vi "Error Handler.vi"(8 "error in":errorcluster, 11 "Engine in":refnum<class "Engine.lvclass">) -> (0 "error out":errorcluster, 2 "Stop Application":bool, 3 "Engine out":refnum<class "Engine.lvclass">)   [LabVIEW 2019, in "Engine.lvclass"]
uses:
  Engine.lvclass
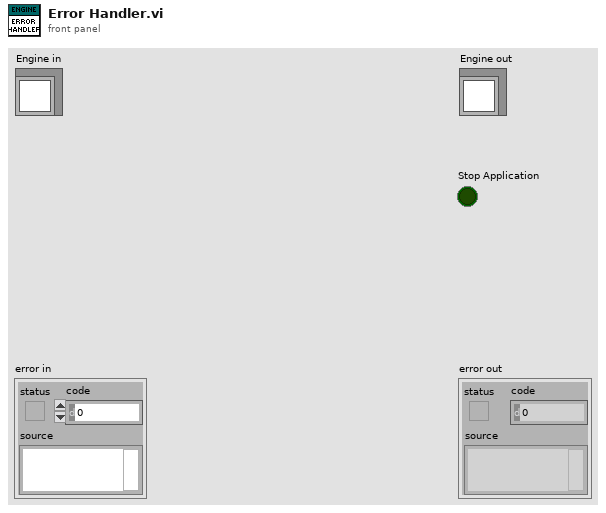
[diagram p1: front panel]
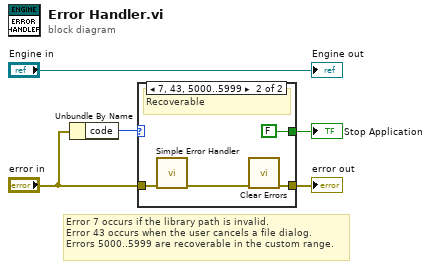
[diagram p0: block diagram]
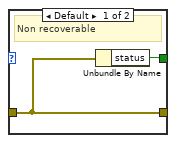
[diagram p2: hidden frame]
diagram:
  # "Error 7 occurs if the library path is invalid.\nError 43 occurs when the user cancels a file dialog.\nErrors 5000..5999 are recoverable in the custom range."
  n1 = Unbundle By Name("error in") -> ("code"=w2:i32)
  n2 = case shown="7, 43, 5000..5999" w2 {
    tunnel: "error in" -> [w7 w11]
    tunnel: [w7 w8] -> w4
    tunnel: [w6 FALSE] -> w1
    frame Default {
      # "Non recoverable"
      n3 = Unbundle By Name(w7) -> ("status"=w6:bool)
    }
    frame 7, 43, 5000..5999 {
      # "Recoverable"
      n4 = call <vilib>:"Simple Error Handler.vi"("error in (no error)"=w11) -> ("error out"=w9:errorcluster)  [unwired: 4 in, 4 out]
      n5 = call <vilib>:"Clear Errors.vi"("error in (no error)"=w9) -> ("error out"=w8:errorcluster)  [unwired: 5 in, 1 out]
    }
  }
  "error out" <- w4
  "Stop Application" <- w1
  "Engine out" <- "Engine in"
